vi "Demo.vi"   [LabVIEW 2021, in "MultiStokePlotDemo.lvlib"]
uses:
  MultiStokePlotDemo.lvlib
  <userlib>/bjustice/RocketPlot/Classes/RocketPlotHandle/SubVIs/Init Options.ctl
  <userlib>/bjustice/RocketPlot/TypeDefs/TimeZone.ctl
  <userlib>/bjustice/RocketPlot/Demo/SubVIs/ring buffer data.ctl
  <userlib>/bjustice/RocketPlot/Classes/NIringPlotHandle/NIringPlotHandle.lvclass
  C:/Program Files/National Instruments/LabVIEW 2021/user.lib/bjustice/RocketPlot/Classes/RocketPlotHandle/RocketPlotHandle.lvclass
  Classes/MultiPlotPanel/MultiPlotPanel.lvclass
  C:/Program Files/National Instruments/LabVIEW 2021/vi.lib/IlluminatedG/IG OOPanel/OOPanel/Panel/Panel.lvclass
  <vilib>/National Instruments/Variant Ring Buffer/Ring Buffer.lvclass
  <vilib>/IlluminatedG/IG OOPanel/OOPanel/Manager/Manager.lvclass
  <userlib>/bjustice/RocketPlot/Demo/RocketPlotDemo.lvlib
  <userlib>/bjustice/RocketPlot/RocketPlot.lvlib
  <userlib>/bjustice/RocketPlot/Classes/RocketPlotHandle/RocketPlotHandle.lvclass
  <userlib>/bjustice/RocketPlot/Classes/RocketPlotPanel/RocketPlotPanel.lvclass
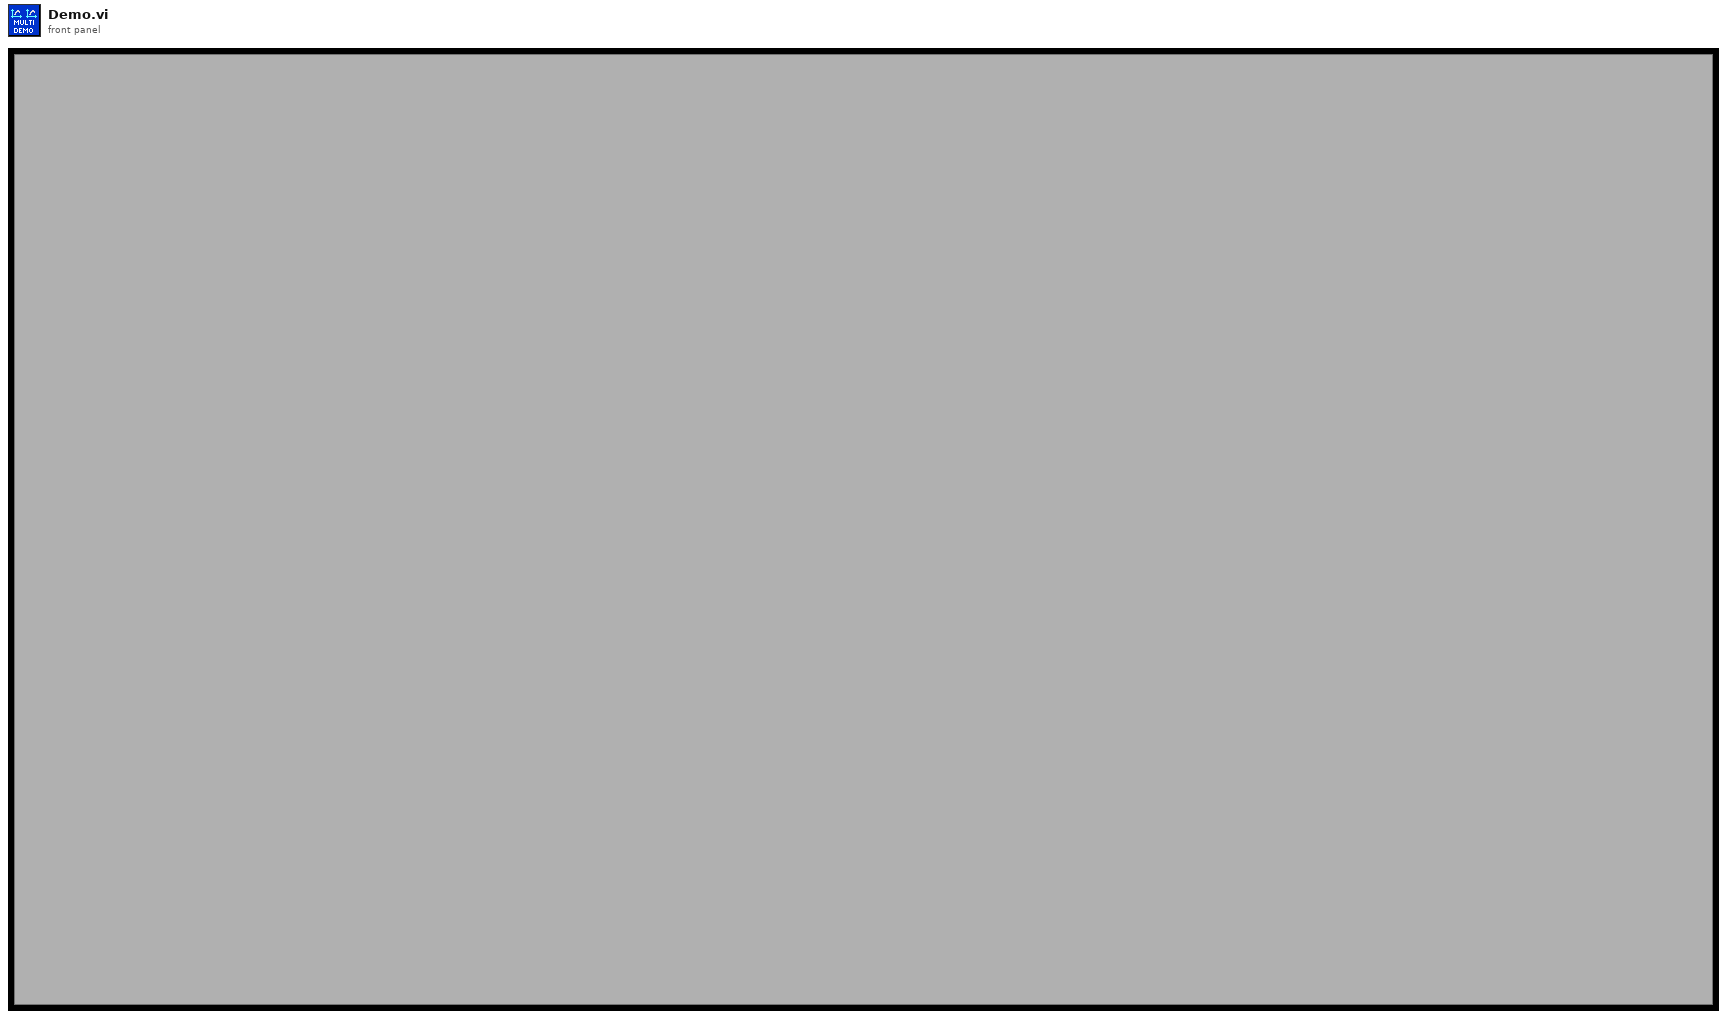
[diagram p1: front panel]
types:
  T1 = typedef "RocketPlotHandle.lvclass/Init Options.ctl" = cluster{"UI visible?":bool, "Update rate (ms)":u32, "Sidebar.Visible":bool, "time to plot (init)":dbl, "time to plot (max)":dbl, "config file start path":path, "Title.Visible":bool, "Title":string, "TimeZone":T2}
  T2 = typedef "RocketPlot.lvlib/TimeZone.ctl" = enum16{"UTC", "Local"}
  T3 = typedef "RocketPlotDemo.lvlib/ring buffer data.ctl" = cluster{"timestamp":dbl, "value":dbl}
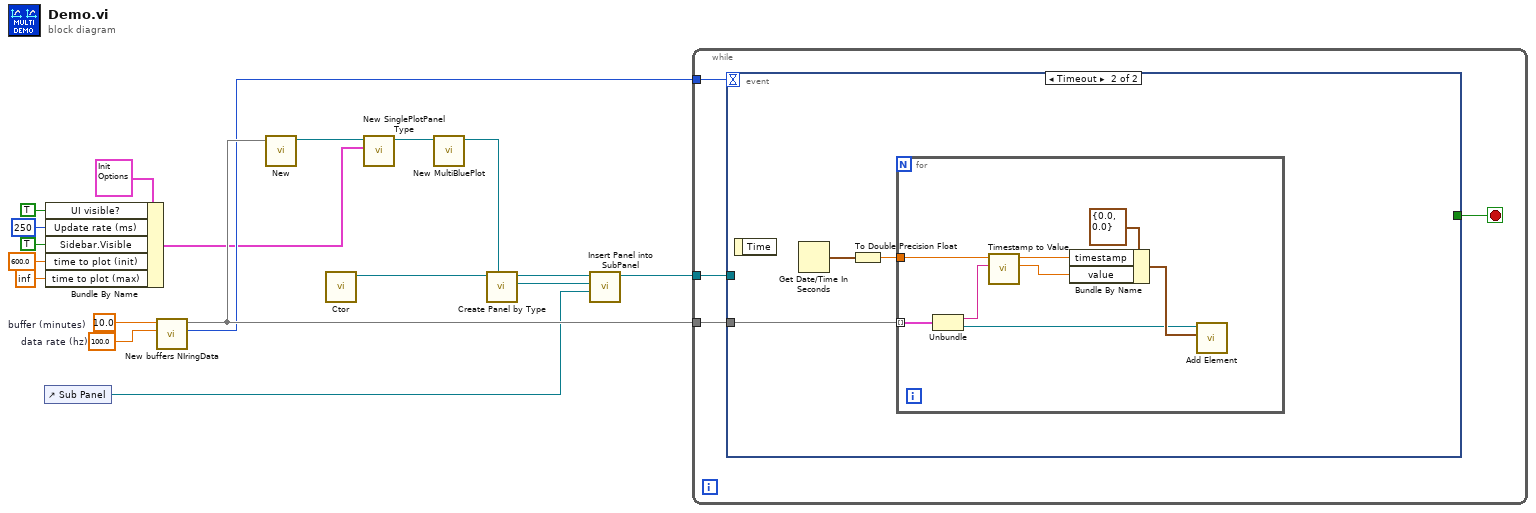
[diagram p0: block diagram]
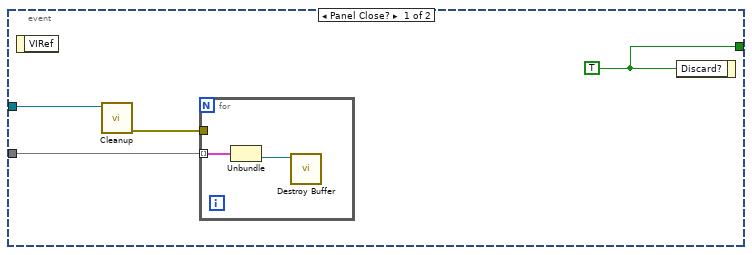
[diagram p2: hidden frame]
diagram:
  w18 = 100.0  # data rate (hz)
  w19 = 10.0  # buffer (minutes)
  n1 = control-ref of="Sub Panel"() -> (w4:refnum<vi>)
  n2 = Bundle By Name(cluster=T1 {"UI visible?"=TRUE, "Update rate (ms)"=250, "Sidebar.Visible"=TRUE, "time to plot (init)"=600.0, "time to plot (max)"=inf, "config file start path"=path "", "Title.Visible"=TRUE, "Title"="Title", "TimeZone"=enum."Local"} ("Init options"), "UI visible?"=TRUE, "Update rate (ms)"=u32 250, "Sidebar.Visible"=TRUE ("visible sidebar?"), "time to plot (init)"=600.0, "time to plot (max)"=inf) -> (w3:T1)
  n3 = call <userlib>:"New buffers NIringData.vi"("data rate (hz)"=w18, "buffer (minutes)"=w19) -> ("period (ms)"=w16:i32, "ChannelMap"=w17:map{string, refnum<data-value>})  [unwired: 8 in]
  n4 = call <userlib>:"New.vi"("ChannelMap"=w17) -> ("plot handle"=w9:refnum<class "NIringPlotHandle.lvclass">)  [unwired: 9 in, 1 out]
  n5 = call <vilib>:"Ctor.vi"() -> ("Manager out"=w8:refnum<class "Manager.lvclass">)  [unwired: 10 in, 1 out]
  n6 = call <userlib>:"New SinglePlotPanel Type.vi"("Init options"=w3, "BluePlotHandle"=w9) -> ("SinglePlotPanel out"=w1:refnum<class "RocketPlotPanel.lvclass">)  [unwired: 8 in, 1 out]
  n7 = call "New MultiBluePlot.vi"("RocketPlotPanel"=w1) -> ("MultiPlotPanel (type)"=w2:refnum<class "MultiPlotPanel.lvclass">)  [unwired: 9 in, 1 out]
  n8 = call <vilib>:"Create Panel by Type.vi"("Panel Type"=w2, "Manager in"=w8) -> ("Panel"=w6:refnum<class "MultiPlotPanel.lvclass">, "Manager out"=w7:refnum<class "Manager.lvclass">)  [unwired: 7 in, 1 out]
  n9 = call <vilib>:"Insert Panel into SubPanel.vi"("SubPanel"=w4, "Panel In"=w6, "Manager in"=w7) -> ("Manager out"=w5:refnum<class "Manager.lvclass">)  [unwired: 6 in, 2 out]
  n10 = while {
    tunnel: w17 -> [w22]
    tunnel: w16 -> [w21]
    tunnel: w5 -> [w20]
    stop <- w23 stop-if-true
    n11 = event shown="[1] Timeout" {
      selector: _ -> [_ _]
      dyn-events: _ -> [_ _]
      timeout: w21 -> [_ _]
      tunnel: [w26 _] -> w23
      tunnel: w22 -> [w27 w32]
      tunnel: w20 -> [w25 _]
      event Panel Close? {
        w26 = TRUE ("Discard?")
        n12 = event-data() -> ()  [unwired: 1 in, 1 out]
        n13 = call <vilib>:"Cleanup.vi"("Manager in"=w25) -> ("error out"=w24:errorcluster)  [unwired: 8 in, 2 out]
        n14 = for {
          tunnel: w24 -> [_]
          tunnel: w27 -> [w29] mode=indexing
          n15 = Unbundle(w29) -> ("Ring Buffer"=w28:refnum<data-value>)  [unwired: 1 out]
          n16 = call <vilib>:"Destroy Buffer.vi"("Ring Buffer Reference"=w28) -> ()  [unwired: 9 in, 2 out]
        }
        n17 = event-data("Discard?"=w26) -> ()  [unwired: 1 in, 1 out]
      }
      event Timeout {
        n18 = event-data() -> ()  [unwired: 1 in, 1 out]
        n19 = Get Date/Time In Seconds() -> (seconds since 1Jan1904=w31:timestamp)
        n20 = To Double Precision Float(number=w31) -> (double precision float=w30:dbl)
        n21 = for {
          tunnel: w32 -> [w35] mode=indexing
          tunnel: w30 -> [w40]
          n22 = Unbundle(w35) -> ("name"=w34:string, "Ring Buffer"=w33:refnum<data-value>)
          n23 = call <userlib>:"Timestamp to Value.vi"("name"=w34, "timestamp"=w40) -> ("value"=w37:dbl, "timestamp (dup)"=w38:dbl)  [unwired: 8 in]
          n24 = Bundle By Name(cluster=T3 {"timestamp"=0.0, "value"=0.0} ("Cluster"), "timestamp"=w38, "value"=w37) -> (w36:T3)
          n25 = call <vilib>:"Add Element.vi"("Variant"=w36, "Ring Buffer Reference"=w33) -> ()  [unwired: 8 in, 2 out]
        }
      }
    }
  }
